vi "Get JSON For Caption and Label.vi"(6 "Force Hide":bool, 8 "error in (no error)":errorcluster, 9 "Evaluate Pane Move":bool, 10 "Data":T1, 11 "VI in":refnum<vi>) -> (0 "error out":errorcluster, 3 "JSON":string)   [LabVIEW 2017, in "Front Panel Publisher.lvlib" / "Control.lvclass"]
doc: "This VI will get the JSON text for any control labels or captions. If the control owning the text is not visible, the text in the JSON string will be blank."
uses:
  Control.lvclass
  Text_class/Text.lvclass
  Attributes.ctl
  Web Front Panel_class/Controls/Enum - Control Display Mode.ctl
  Web Front Panel_class/Web Front Panel.lvclass
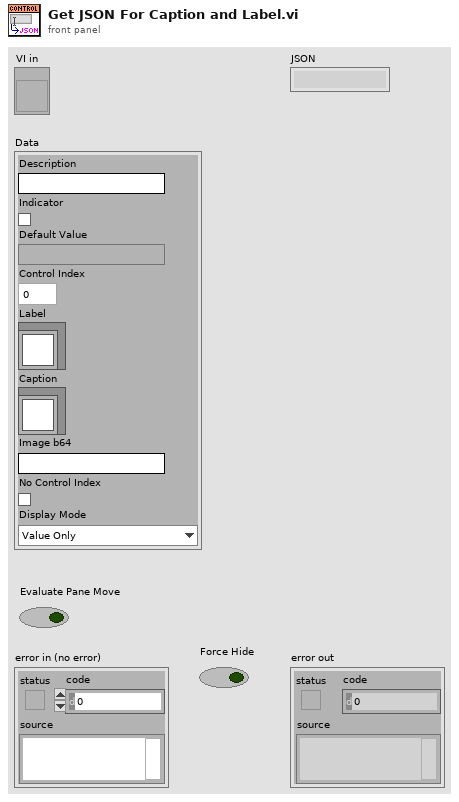
[diagram p1: front panel]
types:
  T1 = typedef "Front Panel Publisher.lvlib/Control.lvclass/Attributes.ctl" = cluster{"Description":string, "Indicator":bool, "Default Value":variant, "Control Index":i32, "Label":refnum<class "Text.lvclass">, "Caption":refnum<class "Text.lvclass">, "Image b64":string, "No Control Index":bool, "Display Mode":T2}
  T2 = typedef "Front Panel Publisher.lvlib/Web Front Panel.lvclass/Enum - Control Display Mode.ctl" = enum16{"Value Only", "Value and Visibility", "Boolean Value Only", "Boolean Value and Visibility", "Control is Image", "Image and Visibility"}
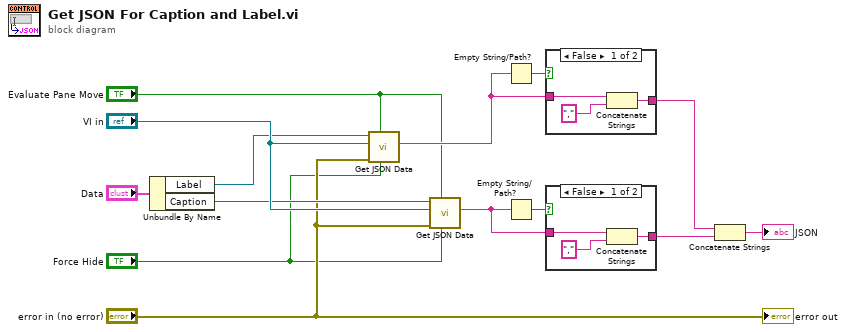
[diagram p0: block diagram]
diagram:
  n1 = Unbundle By Name("Data") -> ("Label"=w12:refnum<class "Text.lvclass">, "Caption"=w13:refnum<class "Text.lvclass">)
  n2 = call-dynamic "Get JSON Data.vi"("Force Hide"="Force Hide", "Evaluate Pane Move"="Evaluate Pane Move", "error in (no error)"="error in (no error)", "VI Reference"="VI in", "Text In"=w12) -> ("JSON string"=w8:string)  [unwired: 4 in, 2 out]
  n3 = call-dynamic "Get JSON Data.vi"("Force Hide"="Force Hide", "Evaluate Pane Move"="Evaluate Pane Move", "error in (no error)"="error in (no error)", "VI Reference"="VI in", "Text In"=w13) -> ("JSON string"=w6:string)  [unwired: 4 in, 2 out]
  n4 = Empty String/Path?(string/path=w8) -> (empty?=w9:bool)
  n5 = Empty String/Path?(string/path=w6) -> (empty?=w7:bool)
  n6 = case shown="False" w9 {
    tunnel: w8 -> [w17 w18]
    tunnel: [w15 w18] -> w3
    frame False {
      n7 = Concatenate Strings(w17, "," ("string")) -> (w15:string)
    }
    frame True {
    }
  }
  n8 = case shown="False" w7 {
    tunnel: w6 -> [w21 w22]
    tunnel: [w19 w22] -> w5
    frame False {
      n9 = Concatenate Strings(w21, "," ("string")) -> (w19:string)
    }
    frame True {
    }
  }
  n10 = Concatenate Strings(w3, w5) -> (→"JSON":string)
  "error out" <- "error in (no error)"
